vi "ni5660 Read Averaged Power Spectrum.vi"(0 "receiver info in":T2, 5 "number of averages":i32=10 min=1, 7 "averaging weighting type":string(combo)="linear", 9 "correction factor":T1[](array[typedef]) {"spectrum correction"."correction factors" format="%.2f"; "spectrum correction"."df" format="%.2f"; "spectrum correction"."f0" format="%.2f"}, 11 "error in (no error)":errorcluster) -> (4 "receiver info out":T2, 6 "averaged power spectrum":cluster{"f0":dbl, "df":dbl, "spectrum":dbl[]}={"f0"=0.0, "df"=1.0, "spectrum"=[]} {"spectrum" format="%.2f"; "df" format="%.2f"; "f0" format="%.2f"}, 8 "spectral info out":T3={"spectrum type"=enum."Power [Magnitude^2]", "linear/dB"=enum."linear", "window"=0, "window size"=1024, "FFT size"=1024} {"window" items=["None ", "Hanning", "Hamming", "Blackman-Harris", "Exact Blackman", "Blackman", "Flat Top", "4 Term B-Harris ", "7 Term B-Harris", "Low Sidelobe"]}, 15 "error out":errorcluster)   [LabVIEW 2011]
doc: "This VI computes the averaged power spectrum that corresponds to the spectral settings specified in the ni5660 Configure for Spectrum VI. The VI returns a cluster that contains the averaged power spectrum in V2rms, starting at frequency <B>f0</B> and frequency interval <B>df</B>. You can perform RMS averaging with linear, exponential, or peak-hold weighting."
uses:
  <vilib>/measure/masml.llb/ma_sml_Spectral Info.ctl
  <vilib>/addons/Modulation/niScope/controls/mod_Modulation Settings.ctl
  <vilib>/addons/Spectral Measurements Toolset/LVSupport/SMT niScope Utilities/smt_correction.ctl
  <vilib>/measure/masml.llb/ma_sml_Averaging Parameters.ctl
  <vilib>/measure/masml.llb/ma_sml_Averaging Settings.ctl
  <vilib>/addons/Spectral Measurements Toolset/LVSupport/SMT niScope Utilities/smt_Apply Correction(power).vi
  <vilib>/addons/Spectral Measurements Toolset/SMT Zoom Power Spectrum for niScope.vi
  <vilib>/addons/Spectral Measurements Toolset/LVSupport/SMT niScope Utilities/smt_Apply Correction(FFT).vi
  <vilib>/measure/NI_MAPro.lvlib
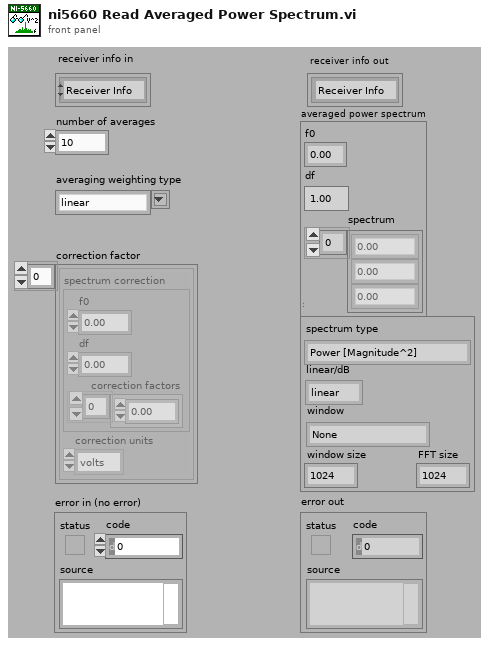
[diagram p1: front panel]
types:
  T1 = typedef "smt_correction.ctl" = cluster{"spectrum correction":cluster{"f0":dbl, "df":dbl, "correction factors":dbl[]}, "correction units":enum16{"volts", "watts", "dB"}}
  T2 = typedef "mod_Modulation Settings.ctl" = cluster{enum16{"Receiver Info"}, variant}
  T3 = typedef "NI_MAPro.lvlib/ma_sml_Spectral Info.ctl" = cluster{"spectrum type":enum16{"FFT Spectrum [complex]", "Amplitude [Magnitude]", "Power [Magnitude^2]", "Cross Spectrum [complex]", "Frequency Response [Complex]"}, "linear/dB":enum16{"linear", "dB"}, "window":u16, "window size":i32, "FFT size":i32}
  T4 = typedef "NI_MAPro.lvlib/ma_sml_Averaging Parameters.ctl" = cluster{"averaging type":enum16{"no averaging", "vector averaging", "RMS averaging", "peak hold"}, "averaging settings":T5}
  T5 = typedef "NI_MAPro.lvlib/ma_sml_Averaging Settings.ctl" = cluster{"weighting type":enum16{"linear", "exponential"}, "weighting settings":cluster{"size":dbl, "linear weighting mode":enum16{"one shot", "auto restart one shot", "moving average", "continuous"}}}
  T6 = enum16{"no averaging", "vector averaging", "RMS averaging", "peak hold"}
  T7 = cluster{"units":enum16{"V", "V^2", "W", "dBm", "dBW", "dBV", "dBmV", "dBuV"}, "peak scaling":enum16{"rms", "pk"}, "psd?":bool, "impedance(ohm)":dbl}
  T8 = enum16{"V", "V^2", "W", "dBm", "dBW", "dBV", "dBmV", "dBuV"}
  T9 = typedef "mod_Readable Attributes Cluster.ctl" = cluster{"carrier":cluster{"frequency":dbl}, "receiver":cluster{"handles":cluster{"niTuner taskID":i32, "niScope handle":refnum<k15>}, "RFSA":cluster{"reference level":i32, "RF attenuation":i32}, "data format":enum16{"real", "complex modulated (array)", "complex modulated (interleaved)"}, "auto suppress SW IQ":enum16{"off", "on"}, "IQ sample rate":dbl, "bandwidth":dbl}}
  T10 = cluster{"multispan?":bool, "segment size":dbl, "number of segments":i32, "frequency shifts":dbl[], "fc adjustment":dbl, "df":dbl, "start frequency (Hz)":dbl, "stop frequency (Hz)":dbl}
  T11 = typedef "NI_MAPro.lvlib/ma_sml_ND Zoom FFT Settings.ctl" = cluster{"zoom settings":cluster{"center frequency":dbl, "zoom":i32, "trim":dbl}, "FFT settings":cluster{"window":u16, "FFT size":i32}}
  T12 = cluster{"zoom FFT settings":T11, "frequency shift":dbl, "data format":enum16{"real", "complex modulated (array)", "complex modulated (interleaved)"}}
  T13 = cluster{"relativeInitialX":dbl, "xIncrement":dbl, "wfm":dbl[]}[]
  T14 = typedef "NI_MAPro.lvlib/ma_sml_Spectrum Cluster (real).ctl" = cluster{"f0":dbl, "df":dbl, "spectrum":dbl[]}
  T15 = cluster{"spectrum type":enum16{"FFT Spectrum [complex]", "Amplitude [Magnitude]", "Power [Magnitude^2]", "Cross Spectrum [complex]", "Frequency Response [Complex]"}, "linear/dB":enum16{"linear", "dB"}, "window":enum16{"None ", "Hanning", "Hamming", "Blackman-Harris", "Exact Blackman", "Blackman", "Flat Top", "4 Term B-Harris ", "7 Term B-Harris", "Low Sidelobe"}, "window size":i32, "FFT size":i32}
  T16 = enum16{"FFT Spectrum [complex]", "Amplitude [Magnitude]", "Power [Magnitude^2]", "Cross Spectrum [complex]", "Frequency Response [Complex]"}
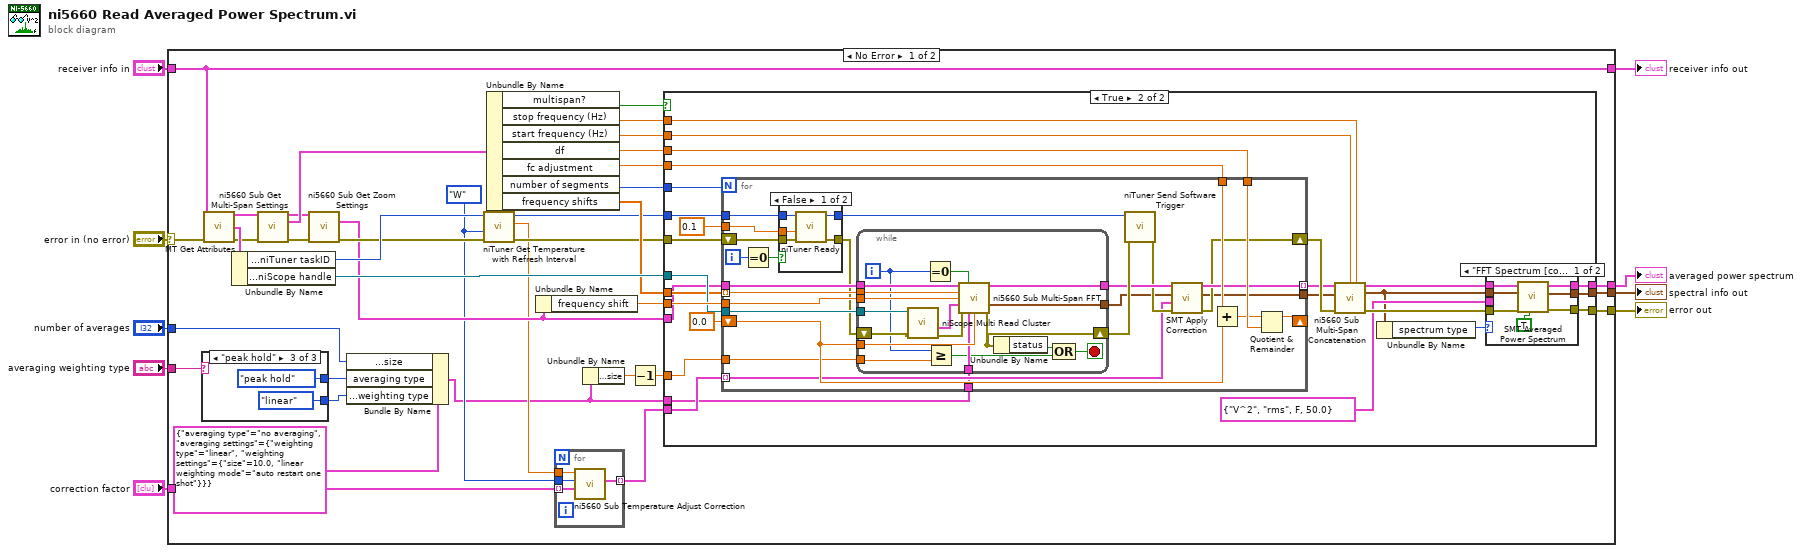
[diagram p0: block diagram]
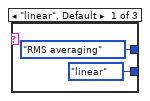
[diagram p2: hidden frame]
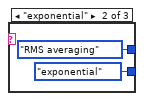
[diagram p3: hidden frame]
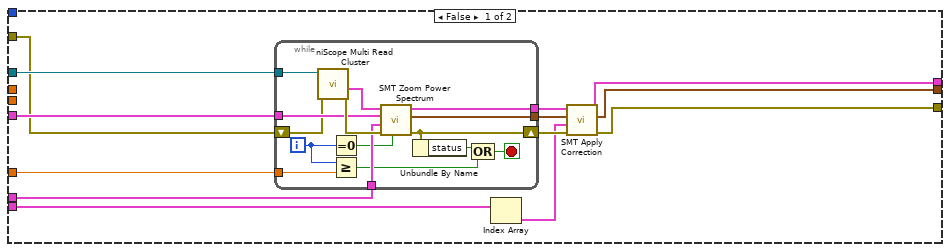
[diagram p4: hidden frame]
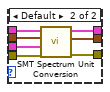
[diagram p5: hidden frame]
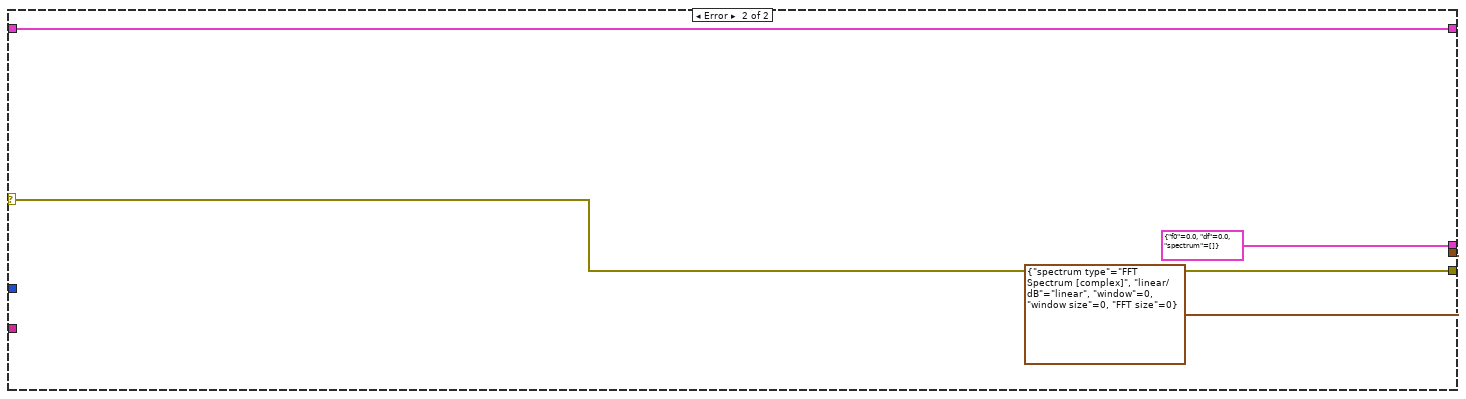
[diagram p7: hidden frame]
diagram:
  n1 = case shown="No Error" "error in (no error)" {
    selector: "error in (no error)" -> [w39 w180]
    tunnel: [w46 w180] -> w9
    tunnel: "correction factor" -> [w45 _]
    tunnel: [w44 cluster{"f0":dbl, "df":dbl, "spectrum":dbl[]} {"f0"=0.0, "df"=0.0, "spectrum"=[]} ("corrected power spectrum")] -> w3
    tunnel: [w43 T3 {"spectrum type"=enum."FFT Spectrum [complex]", "linear/dB"=enum."linear", "window"=0, "window size"=0, "FFT size"=0} ("spectral info out")] -> w7
    tunnel: "receiver info in" -> [w38 w179]
    tunnel: [w38 w179] -> w5
    tunnel: "averaging weighting type" -> [w17 _]
    tunnel: "number of averages" -> [w14 _]
    frame No Error {
      w19 = T8."W" ("correction units")
      n2 = case shown="\"peak hold\"" w17 {
        tunnel: [T6."RMS averaging" ("averaging type") T6."RMS averaging" ("averaging type") T6."peak hold" ("averaging type")] -> w15
        tunnel: [enum16{"linear", "exponential"}."linear" ("weighting type") enum16{"linear", "exponential"}."exponential" ("weighting type") enum16{"linear", "exponential"}."linear" ("weighting type")] -> w13
        frame "linear", Default {
        }
        frame "exponential" {
        }
        frame "peak hold" {
        }
      }
      n3 = call <vilib>:"MT Get Attributes.vi"("receiver info in"=w38, "error in (no error)"=w39) -> ("receiver info out"=w37:T2, "attributes"=w42:T9, "error out"=w36:errorcluster)  [unwired: 11 in]
      n4 = Unbundle By Name(w42) -> ("receiver.handles.niTuner taskID"=w40:i32, "receiver.handles.niScope handle"=w41:refnum<k15>)
      n5 = call <instrlib>:"ni5660 Sub Get Multi-Span Settings.vi"("receiver info in"=w37, "error in (no error)"=w36) -> ("receiver info out"=w33:T2, "multispan settings"=w35:T10, "error out"=w34:errorcluster)  [unwired: 10 in, 1 out]
      n6 = call <instrlib>:"ni5660 Sub Get Zoom Settings.vi"("receiver info in"=w33, "error in (no error)"=w34) -> ("zoom settings"=w31:T12, "error out"=w32:errorcluster)  [unwired: 10 in, 2 out]
      n7 = Bundle By Name(cluster=T4 {"averaging type"=enum."no averaging", "averaging settings"={"weighting type"=enum."linear", "weighting settings"={"size"=10.0, "linear weighting mode"=enum."auto restart one shot"}}} ("averaging parameters"), "averaging settings.weighting settings.size"=w14, "averaging type"=w15, "averaging settings.weighting type"=w13) -> (w12:T4)
      n8 = call <instrlib>:"niTuner Get Temperature with Refresh Interval.vi"("error in"=w32, "correction units"=w19, "taskID in"=w40) -> ("error out"=w21:errorcluster, "correction factor"=w20:dbl, "taskID out"=w22:i32)  [unwired: 5 in, 1 out]
      n9 = Unbundle By Name(w35) -> ("multispan?"=w23:bool, "stop frequency (Hz)"=w24:dbl, "start frequency (Hz)"=w29:dbl, "df"=w28:dbl, "fc adjustment"=w27:dbl, "number of segments"=w18:i32, "frequency shifts"=w26:dbl[])
      n10 = Unbundle By Name(w31) -> ("frequency shift"=w30:dbl)
      n11 = for {
        tunnel: [w56] -> w25 mode=indexing
        tunnel: w45 -> [w55] mode=indexing
        tunnel: w20 -> [w54]
        tunnel: w19 -> [w53]
        n12 = call <instrlib>:"ni5660 Sub Temperature Adjust Correction.vi"("correction"=w55, "temperature correction units"=w53, "temperature correction factor"=w54) -> ("temperature adjusted correction"=w56:T1)  [unwired: 8 in]
      }
      n13 = Unbundle By Name(w12) -> ("averaging settings.weighting settings.size"=w11:dbl)
      n14 = Decrement(x=w11) -> (x-1=w10:dbl)
      n15 = case shown="True" w23 {
        tunnel: w30 -> [_ w111]
        tunnel: w41 -> [w69 w106]
        tunnel: w29 -> [_ w105]
        tunnel: w28 -> [_ w104]
        tunnel: w27 -> [_ w103]
        tunnel: w26 -> [_ w102]
        tunnel: w25 -> [w65 w101]
        tunnel: [w63 w94] -> w46
        tunnel: w24 -> [_ w100]
        tunnel: [w60 w93] -> w44
        tunnel: [w64 w92] -> w43
        tunnel: w21 -> [w59 w90]
        tunnel: w22 -> [_ w89]
        tunnel: w31 -> [w61 w99]
        tunnel: w12 -> [w58 w98]
        tunnel: w18 -> [_ w97]
        tunnel: w10 -> [w57 w85]
        frame False {
          n16 = while {
            tunnel: w69 -> [w84]
            tunnel: [w82] -> w68
            tunnel: [w81] -> w67
            tunnel: w61 -> [w80]
            shift-right: [w78] -> w66
            shift-left: w59 -> [w79]
            tunnel: w58 -> [w75]
            tunnel: w57 -> [w71]
            i -> [w73]
            stop <- w76 stop-if-true
            n17 = call <instrlib>:"niScope Multi Read Cluster.vi"("error in"=w79, "instrument handle"=w84) -> ("error out"=w83:errorcluster, "waveform"=w77:T13)  [unwired: 6 in, 2 out]
            n18 = Equal To 0?(x=w73) -> (x = 0?=w74:bool)
            n19 = Greater Or Equal?(x=w73, y=w71) -> (x >= y?=w70:bool)
            n20 = call-poly <vilib>:"SMT Zoom Power Spectrum.vi"("restart averaging?"=w74, "error in (no error)"=w83, "averaging parameters"=w75, "SMT zoom settings"=w80, "waveforms"=w77) -> ("error out"=w78:errorcluster, "spectral info"=w81:T3, "power spectrum"=w82:T14)  [unwired: 2 in, 2 out]
            n21 = Unbundle By Name(w78) -> ("status"=w72:bool)
            n22 = Compound Arithmetic op=OR(w72, w70) -> (w76:bool)
          }
          n23 = Index Array(array=w65) -> (element=w62:T1)  [unwired: 1 in]
          n24 = call-poly <vilib>:"SMT Apply Correction.vi"("error in (no error)"=w66, "correction"=w62, "spectral info in"=w67, "power spectrum"=w68) -> ("error out"=w63:errorcluster, "spectral info out"=w64:T3, "corrected power spectrum"=w60:cluster{"f0":dbl, "df":dbl, "spectrum":dbl[]})  [unwired: 5 in]
        }
        frame True {
          n25 = for {
            N: w97 -> [_]
            tunnel: w106 -> [w145]
            tunnel: [w135] -> w108
            tunnel: w102 -> [w143] mode=indexing
            shift-right: [w146] -> _
            shift-left: 0.0 ("timeout") -> [w141]
            tunnel: w103 -> [w150]
            tunnel: w104 -> [w151]
            shift-right: [w136] -> w110
            shift-left: w90 -> [w147]
            tunnel: w99 -> [w144]
            tunnel: w111 -> [w142]
            tunnel: w101 -> [w134] mode=indexing
            tunnel: [w137] -> w107 mode=indexing
            tunnel: w98 -> [w131]
            tunnel: w89 -> [w130]
            tunnel: 0.1 ("timeout") -> [w129]
            tunnel: w85 -> [w126]
            i -> [w128]
            n26 = Equal To 0?(x=w128) -> (x = 0?=w127:bool)
            n27 = case shown="False" w127 {
              tunnel: [w156 w157] -> w148
              tunnel: w147 -> [w155 w158]
              tunnel: [w154 w158] -> w132
              tunnel: w130 -> [w153 w157]
              tunnel: w129 -> [w152 _]
              frame False {
                n28 = call <instrlib>:"niTuner Ready.vi"("error in"=w155, "timeout"=w152, "taskID in"=w153) -> ("error out"=w154:errorcluster, "taskID out"=w156:i32)  [unwired: 6 in, 1 out]
              }
              frame True {
              }
            }
            n29 = while {
              tunnel: w145 -> [w176]
              shift-right: [w165] -> w140
              shift-left: w132 -> [w175]
              tunnel: w144 -> [w174]
              tunnel: w143 -> [w172]
              tunnel: w142 -> [w171]
              tunnel: w141 -> [w169]
              tunnel: [w168] -> w139
              tunnel: [w167] -> w133
              tunnel: w131 -> [w164]
              tunnel: w126 -> [w159]
              i -> [w161]
              stop <- w166 stop-if-true
              n30 = call <instrlib>:"niScope Multi Read Cluster.vi"("error in"=w175, "instrument handle"=w176) -> ("error out"=w173:errorcluster, "waveform"=w163:T13)  [unwired: 6 in, 2 out]
              n31 = Equal To 0?(x=w161) -> (x = 0?=w170:bool)
              n32 = Greater Or Equal?(x=w161, y=w159) -> (x >= y?=w160:bool)
              n33 = call <instrlib>:"ni5660 Sub Multi-Span FFT.vi"("SMT zoom settings"=w174, "restart averaging?"=w170, "Tuner Frequency Shift"=w172, "DDC Frequency Shift"=w171, "waveform"=w163, "error in (no error)"=w173, "averaging parameters"=w164, "fc adjust"=w169) -> ("averaged FFT spectrum"=w168:cluster{"f0":dbl, "df":dbl, "spectrum":cdb[]}, "spectral info in"=w167:T15, "error out"=w165:errorcluster)  [unwired: 3 in, 2 out]
              n34 = Unbundle By Name(w165) -> ("status"=w162:bool)
              n35 = Compound Arithmetic op=OR(w162, w160) -> (w166:bool)
            }
            n36 = call <instrlib>:"niTuner Send Software Trigger.vi"("error in"=w140, "taskID in"=w148) -> ("error out"=w138:errorcluster)  [unwired: 8 in, 1 out]
            n37 = call-poly <vilib>:"SMT Apply Correction.vi"("error in (no error)"=w138, "correction"=w134, "spectral info in"=w133, "FFT spectrum"=w139) -> ("error out"=w136:errorcluster, "spectral info out"=w135:T3, "corrected FFT spectrum"=w137:cluster{"f0":dbl, "df":dbl, "spectrum":cdb[]})  [unwired: 5 in]
            n38 = Add(x=w150, y=w141) -> (x+y=w149:dbl)
            n39 = Quotient & Remainder(x=w149, y=w151) -> (x-y*floor(x/y)=w146:dbl)  [unwired: 1 out]
          }
          n40 = call <instrlib>:"ni5660 Sub Multi-Span Concatenation.vi"("FFT spectrum array"=w107, "Fstart"=w105, "Fstop"=w100, "spectral info in"=w108, "error in (no error)"=w110) -> ("concatenated FFT spectrum"=w96:cluster{"f0":dbl, "df":dbl, "spectrum":cdb[]}, "spectral info out"=w87:T3, "error out"=w95:errorcluster)  [unwired: 7 in, 1 out]
          n41 = Unbundle By Name(w87) -> ("spectrum type"=w86:T16)
          n42 = case shown="\"FFT Spectrum [complex]\"" w86 {
            tunnel: w96 -> [w118 w125]
            tunnel: w87 -> [w114 w124]
            tunnel: w95 -> [w116 w123]
            tunnel: [w115 w122] -> w94
            tunnel: [w117 w121] -> w93
            tunnel: [w113 w120] -> w92
            tunnel: T7 {"units"=enum."V^2", "peak scaling"=enum."rms", "psd?"=FALSE, "impedance(ohm)"=50.0} ("unit conversion settings") -> [_ w119]
            frame "FFT Spectrum [complex]" {
              n43 = call <vilib>:"SMT Averaged Power Spectrum.vi"("restart averaging?"=TRUE, "error in (no error)"=w116, "spectral info in"=w114, "FFT spectrum"=w118) -> ("error out"=w115:errorcluster, "spectral info out"=w113:T3, "averaged power spectrum"=w117:cluster{"f0":dbl, "df":dbl, "spectrum":cdb[]})  [unwired: 3 in, 2 out]
            }
            frame Default {
              n44 = call <vilib>:"SMT Spectrum Unit Conversion.vi"("error in (no error)"=w123, "unit conversion settings"=w119, "spectral info in"=w124, "power spectrum"=w125) -> ("error out"=w122:errorcluster, "spectral info out"=w120:T3, "unit converted spectrum"=w121:cluster{"f0":dbl, "df":dbl, "spectrum":dbl[]})  [unwired: 4 in, 1 out]
            }
          }
        }
      }
    }
    frame Error {
    }
  }
  "error out" <- w9
  "spectral info out" <- w7
  "receiver info out" <- w5
  "averaged power spectrum" <- w3
